vi "append_file_with_file.vi"() -> ()   [LabVIEW 2014]
uses:
  <vilib>/Utility/NIReport.llb/NI_report.lvclass
panel:
  out "end out (Word)":i32
  out "start out (Word)":i32
  in  "is spreadsheet file? (Excel)":bool
  in  "file path":path
  in  "template (empty)":path
  out "report type":T1(ring)=enum."HTML"
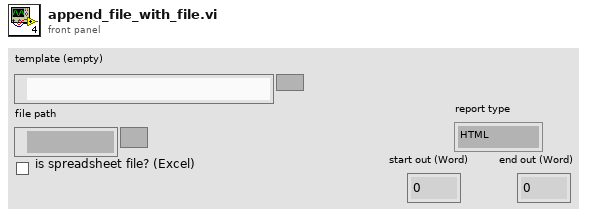
[diagram p1: front panel]
types:
  T1 = enum16{"Standard Report", "HTML", "Word", "Excel"}
  T2 = enum16{"maximized", "minimized", "normal", "no change"}
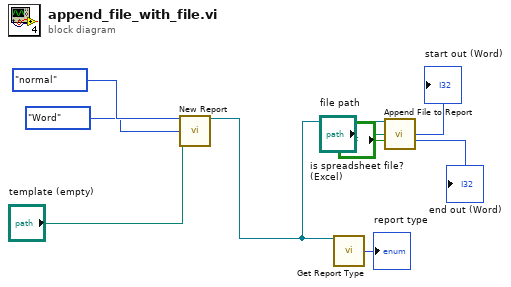
[diagram p0: block diagram]
diagram:
  n1 = call <vilib>:"New Report.vi"("window state (normal)"=T2."normal", "report type"=T1."Word", "template (empty)"="template (empty)") -> ("report out"=w5:refnum<class "NI_report.lvclass">)  [unwired: 11 in, 1 out]
  n2 = call-dynamic "Get Report Type.vi"("report in"=w5) -> ("report type"=→"report type":T1)  [unwired: 12 in, 2 out]
  n3 = call-dynamic "Append File to Report.vi"("report in"=w5, "file path"="file path", "is spreadsheet file? (Excel)"="is spreadsheet file? (Excel)") -> ("start out (Word)"=→"start out (Word)":i32, "end out (Word)"=→"end out (Word)":i32)  [unwired: 9 in, 2 out]
